vi "CC Filter Names from Control Refs.vi"(8 "error in (no error)":errorcluster, 11 "Filter Refs":refnum<vi>[](array[refnum])) -> (0 "error out":errorcluster, 3 "Filter names":string[](array[string]))   [LabVIEW 2024]
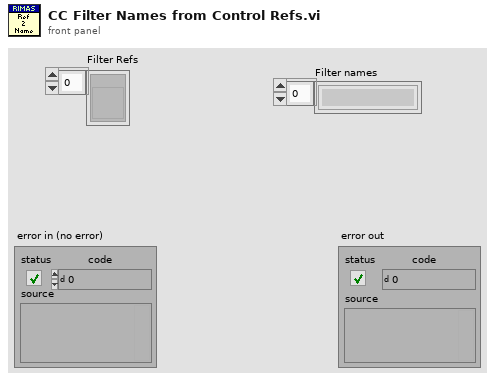
[diagram p1: front panel]
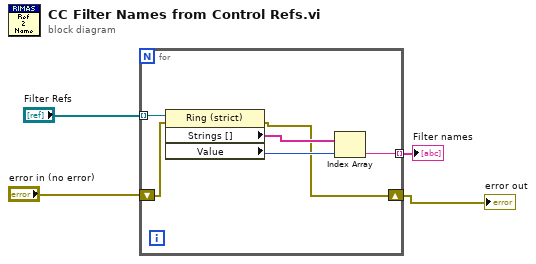
[diagram p0: block diagram]
diagram:
  n1 = for {
    tunnel: "Filter Refs" -> [w10] mode=indexing
    tunnel: [w7] -> w3 mode=indexing
    shift-right: [w5] -> w1
    shift-left: "error in (no error)" -> [w6]
    n2 = property class="Ring (strict)"(reference=w10, error in=w6) -> (error out=w5:errorcluster, "Strings []"=w9:string[], "Value"=w8:u16)  [unwired: 1 out]
    n3 = Index Array(array=w9, index=w8) -> (element=w7:string)
  }
  "error out" <- w1
  "Filter names" <- w3
